vi "CameraAbort.vi"(8 "error in (no error)":errorcluster, 11 "AndorSDK2 in":refnum<class "Andor2.lvclass">) -> (0 "error out":errorcluster, 3 "AndorSDK2 out":refnum<class "Andor2.lvclass">)   [LabVIEW 2010, in "Andor2.lvclass"]
uses:
  Andor2.lvclass
  <userlib>/Andor/atmcd32d.llb/Shutter_mode typedef.ctl
  <userlib>/Andor/atmcd32d.llb/Shutter_type typedef.ctl
  Andor2.lvclass/Andor2.ctl
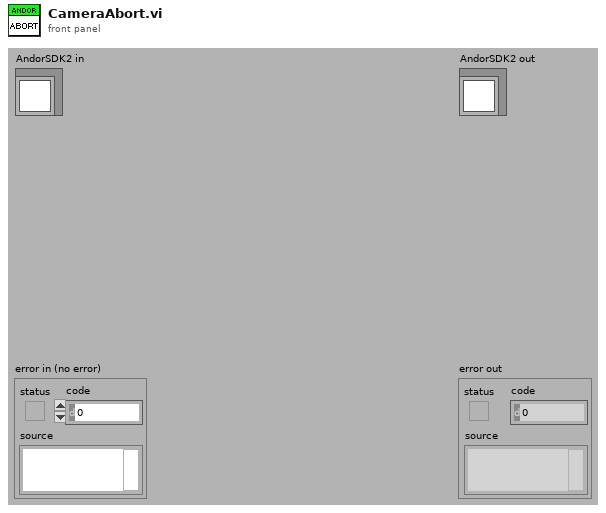
[diagram p1: front panel]
types:
  T1 = typedef "Shutter_mode typedef.ctl" = enum16{"Auto", "Open", "Close"}
  T2 = typedef "Shutter_type typedef.ctl" = enum16{"TTL Low", "TTL High"}
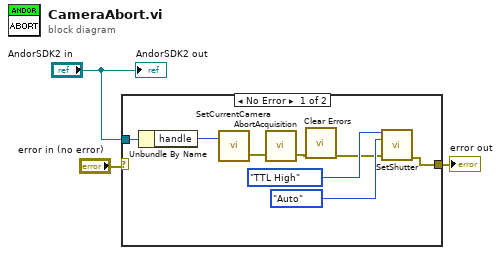
[diagram p0: block diagram]
diagram:
  n1 = case shown="No Error" "error in (no error)" {
    selector: "error in (no error)" -> [_ w12]
    tunnel: "AndorSDK2 in" -> [w9 _]
    tunnel: [w4 w12] -> w1
    frame No Error {
      n2 = Unbundle By Name(w9) -> ("handle"=w11:i32)
      n3 = call <userlib>:"SetCurrentCamera.vi"("cameraHandle"=w11) -> ("error out"=w10:errorcluster)  [unwired: 1 in, 1 out]
      n4 = call <userlib>:"AbortAcquisition.vi"("error in (no error)"=w10) -> ("error out"=w6:errorcluster)  [unwired: 1 in, 1 out]
      n5 = call <vilib>:"Clear Errors.vi"("error in (no error)"=w6) -> ("error out"=w5:errorcluster)  [unwired: 6 in]
      n6 = call <userlib>:"SetShutter.vi"("type"=Shutter_type_typedef."TTL High", "mode"=Shutter_mode_typedef."Auto", "error in (no error)"=w5) -> ("error out"=w4:errorcluster)  [unwired: 11 in, 1 out]
    }
    frame Error {
    }
  }
  "error out" <- w1
  "AndorSDK2 out" <- "AndorSDK2 in"
